vi "Create Network Stream Listener.vi"(6 "Buffer Size":i32=4096, 11 "Name":string) -> (3 "Network Stream Listener":refnum<class "Network Stream Listener.lvclass">)   [LabVIEW 2020, in "Network Stream Listener.lvclass"]
doc: "Use this method to configure a Network Stream Listener for use."
uses:
  Network Stream Listener.lvclass
  Network Stream/Network Stream.lvclass
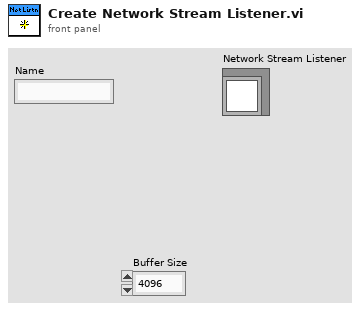
[diagram p1: front panel]
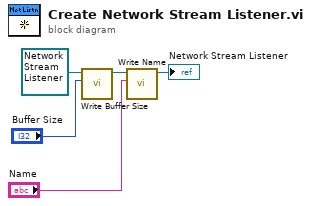
[diagram p0: block diagram]
diagram:
  n1 = call "Write Buffer Size.vi"("Buffer Size"="Buffer Size", "Network Stream in"=refnum<class "Network Stream Listener.lvclass"> refnum ("Network Stream Listener in")) -> ("Network Stream out"=w4:refnum<class "Network Stream Listener.lvclass">)  [unwired: 9 in]
  n2 = call "Write Name.vi"("Name"="Name", "Network Stream in"=w4) -> ("Network Stream out"=→"Network Stream Listener":refnum<class "Network Stream Listener.lvclass">)  [unwired: 9 in]
